vi "I2C Read.vi"(8 "error in (no error)":errorcluster, 9 "Timeout (1000 ms)":u16=1000, 10 "# Bytes to Read":u8, 11 "LINX I2C in":refnum<class "LINX I2C.lvclass">) -> (0 "error out":errorcluster, 2 "Bytes Read":u8[](array[numeric]), 3 "LINX I2C out":refnum<class "LINX I2C.lvclass">)   [LabVIEW 2020, in "LINX I2C.lvclass"]
uses:
  LINX I2C.lvclass
  LINX I2C.lvclass/LINX I2C.ctl
  <vilib>/MakerHub/LINX/LMH-LINX.lvlib
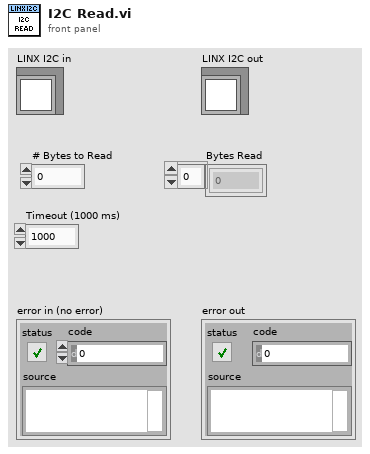
[diagram p1: front panel]
types:
  T1 = typedef "LMH-LINX.lvlib/LINX Ref.ctl" = cluster{"IO":T2, "Interface":T3, "LINX Device Config":T4}
  T2 = typedef "LMH-LINX.lvlib/Platform.ctl" = enum16{"Remote", "Local"}
  T3 = typedef "LMH-LINX.lvlib/Interface.ctl" = enum16{"Serial", "TCP"}
  T4 = typedef "LMH-LINX.lvlib/Device.lvlib/LINX Device Config.ctl" = cluster{"Interface":T3, "COM Port":refnum<visa-resource-name>, "TCP Configuration":T5, "Device Family":u8, "Device ID":u8, "Device Name":string, "TCP Ref":refnum<k5>, "Channels":T6}
  T5 = typedef "LMH-LINX.lvlib/Device.lvlib/TCP Config.ctl" = cluster{"IP Address":string, "Port":u16}
  T6 = typedef "LMH-LINX.lvlib/Channels.ctl" = cluster{"DI":u8[], "DO":u8[], "AI":u8[], "AO":u8[], "PWM":u8[], "QE":u8[], "UART":u8[], "I2C 2":u8[], "SPI":u8[], "CAN":u8[], "Servo":u8[], "AI Ref (V)":dbl, "AI Resolution (Bits)":u8, "AO Ref (V)":dbl, "AO Resolution (Bits)":u8}
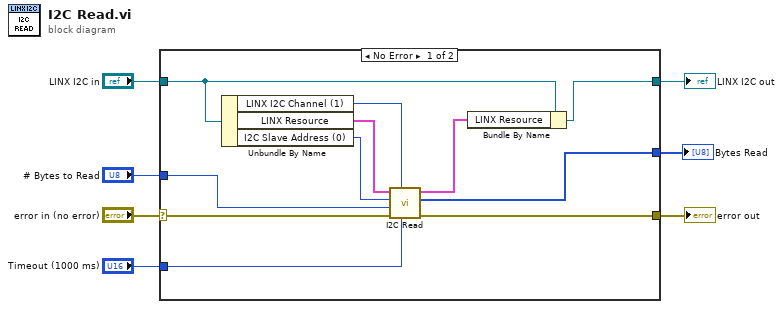
[diagram p0: block diagram]
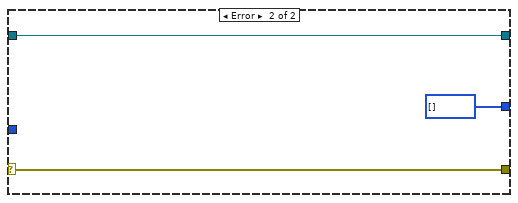
[diagram p2: hidden frame]
diagram:
  n1 = case shown="No Error" "error in (no error)" {
    selector: "error in (no error)" -> [w15 w21]
    tunnel: [w11 w19] -> w7
    tunnel: "LINX I2C in" -> [w12 w19]
    tunnel: [w14 w21] -> w5
    tunnel: "# Bytes to Read" -> [w18 _]
    tunnel: [w17 u8[] [] ("Data")] -> w2
    tunnel: "Timeout (1000 ms)" -> [w16 _]
    frame No Error {
      n2 = Unbundle By Name(w12) -> ("LINX I2C Channel (1)"=w9:u8, "LINX Resource"=w13:T1, "I2C Slave Address (0)"=w8:u8)
      n3 = call <vilib>:"I2C Read.vi"("Timeout (1000 ms)"=w16, "I2C Channel"=w9, "Error In"=w15, "Bytes To Read"=w18, "I2C Slave Address (0)"=w8, "LINX Resource"=w13) -> ("Error Out"=w14:errorcluster, "Data"=w17:u8[], "LINX Resource"=w10:T1)  [unwired: 3 in]
      n4 = Bundle By Name(cluster=w12, "LINX Resource"=w10) -> (w11:refnum<class "LINX I2C.lvclass">)
    }
    frame Error {
    }
  }
  "Bytes Read" <- w2
  "LINX I2C out" <- w7
  "error out" <- w5
